vi "TestExec.Analyze Result and Promote Specified Record.vi"(8 "Demoted Name":string, 9 "Data.MeasData":T1[](array[typedef]) {"Status" items=["LOG", "PASS", "FAIL", "ERROR"]}, 10 "ResultState":T3={"State"=enum."Passing", "Code"=0, "Description"=""}, 11 "TE Q":refnum<queue>) -> ()   [LabVIEW 2018]
uses:
  <vilib>/KATE/Queues/Q.Element.ctl
  Results/Result.Measurement Item.ctl
  Results/Result.Measurement and Attribute Item Status.ctl
  <vilib>/KATE/SeqMgr/SeqMgr.Result Info.ctl
  <vilib>/KATE/SeqMgr/SeqMgr.Result State Enum.ctl
  <vilib>/KATE/SeqMgr/SeqMgr.lvlib
  <vilib>/KATE/Queues/Queue Utils.lvlib
panel:
  out "Data.MeasData Out":T1[](array[typedef]) {"Status" items=["LOG", "PASS", "FAIL", "ERROR"]}
  out "ResultState Out":T3={"State"=enum."Failing", "Code"=0, "Description"=""}
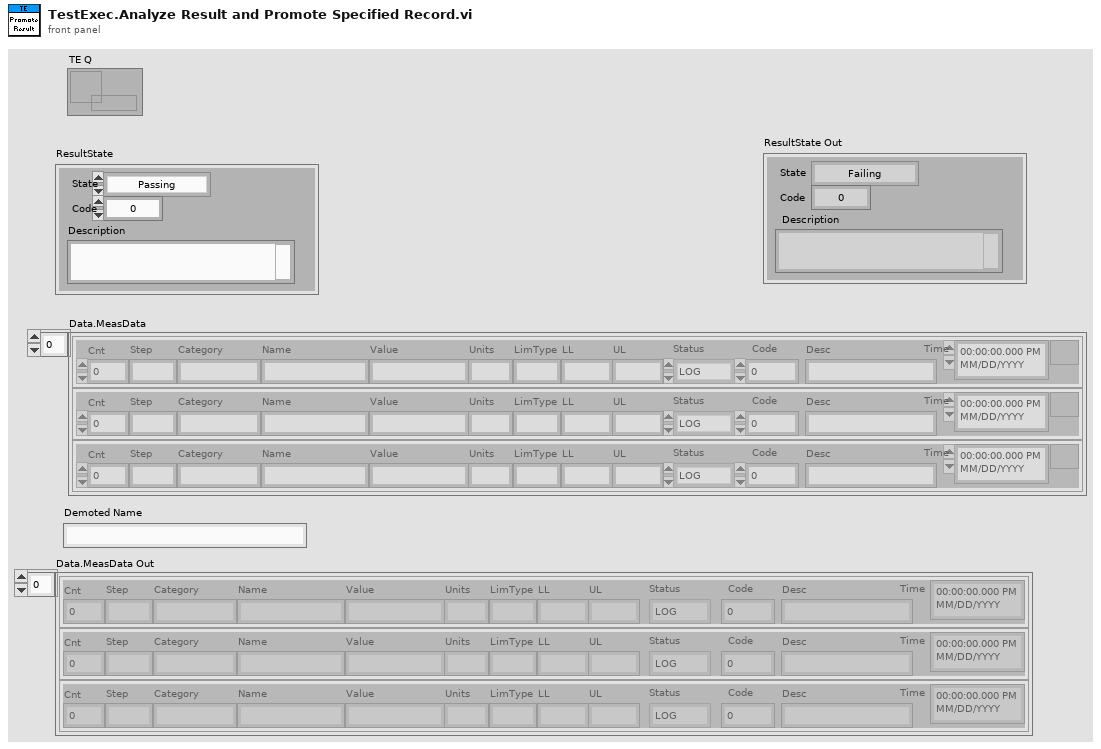
[diagram p1: front panel]
types:
  T1 = typedef "Result.Measurement Item.ctl" = cluster{"Cnt":i32, "Step":string, "Category":string, "Name":string, "Value":string, "Units":string, "LimType":string, "LL":string, "UL":string, "Status":T2, "Code":i32, "Desc":string, "Time":timestamp}
  T2 = typedef "Result.Measurement and Attribute Item Status.ctl" = i32
  T3 = typedef "KATE_Lib.lvlib/SeqMgr.lvlib/SeqMgr.Result Info.ctl" = cluster{"State":T4, "Code":i32, "Description":string}
  T4 = typedef "KATE_Lib.lvlib/SeqMgr.lvlib/SeqMgr.Result State Enum.ctl" = enum16{"None", "Passing", "Failing", "PASS", "FAIL", "ABORT", "ERROR"}
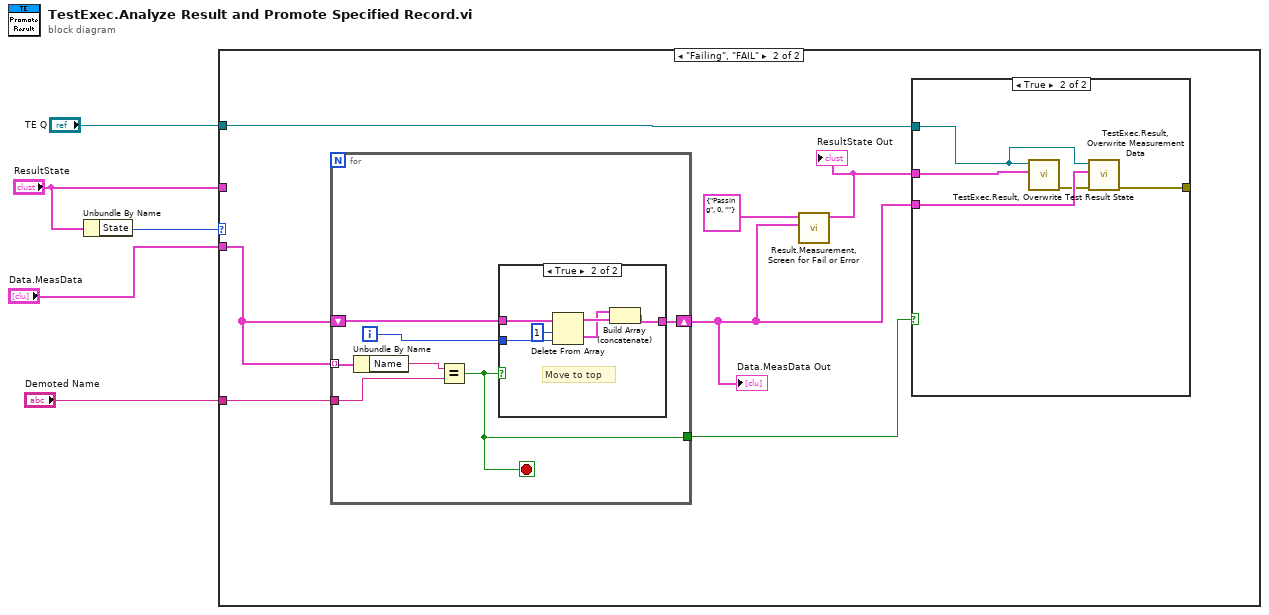
[diagram p0: block diagram]
diagram:
  n1 = Unbundle By Name("ResultState") -> ("State"=w3:T4)
  n2 = case shown="\"Failing\", \"FAIL\"" w3 {
    tunnel: "Data.MeasData" -> [_ w12]
    tunnel: "TE Q" -> [_ w10]
    tunnel: "ResultState" -> [_ _]
    tunnel: "Demoted Name" -> [_ w7]
    frame "None", Default {
    }
    frame "Failing", "FAIL" {
      n3 = for {
        tunnel: w12 -> [w24] mode=indexing
        shift-right: [w20] -> w6
        shift-left: w12 -> [w22]
        tunnel: [w19] -> w11
        tunnel: w7 -> [w18]
        i -> [w21]
        stop <- w19 stop-if-true
        n4 = Unbundle By Name(w24) -> ("Name"=w23:string)
        n5 = Equal?(x=w23, y=w18) -> (x = y?=w19:bool)
        n6 = case shown="True" w19 {
          tunnel: w22 -> [w25 w31]
          tunnel: w21 -> [_ w30]
          tunnel: [w25 w27] -> w20
          frame False {
          }
          frame True {
            # "Move to top"
            n7 = Delete From Array(array=w31, length=1, index=w30) -> (deleted portion=w26:T1[], array with subset deleted=w28:T1[])
            n8 = Build Array (concatenate)(w26, w28) -> (w27:T1[])
          }
        }
      }
      "Data.MeasData Out" <- w6
      n9 = call "Result.Measurement, Screen for Fail or Error.vi"("Meas"=w6, "ResultState In"=T3 {"State"=enum."Passing", "Code"=0, "Description"=""} ("ResultState Out")) -> ("ResultState Out"=w8:T3)  [unwired: 9 in]
      "ResultState Out" <- w8
      n10 = case shown="True" w11 {
        tunnel: w6 -> [_ w16]
        tunnel: w10 -> [_ w17]
        tunnel: w8 -> [_ w15]
        tunnel: [_ w13] -> _
        frame False {
        }
        frame True {
          n11 = call "TestExec.Result, Overwrite Test Result State.vi"("ResultState"=w15, "Q In"=w17) -> ("error out"=w14:errorcluster)  [unwired: 9 in]
          n12 = call "TestExec.Result, Overwrite Measurement Data.vi"("error in"=w14, "Meas Data"=w16, "Q In"=w17) -> ("error out"=w13:errorcluster)  [unwired: 8 in]
        }
      }
    }
  }
